vi "Drive Controller.vi"(8 "error in":errorcluster) -> ()   [LabVIEW 2020]
doc: "This VI executes continuously carrying out the current operation and responding to updates or new operation requests. It will often contain the timing or control code that is difficult to place directly in TeleOp. This VI generally opens all sensors and motors and isolates the rest of the robot code from knowing implementation details of how the operations are carried out."
uses:
  <vilib>/Rock Robotics/WPI/Framework/Completion Status.ctl
  Drive Setpoints.ctl
  Drive Operations.ctl
  <vilib>/Rock Robotics/WPI/SafetyOutput/WPI_SafetyOutputConfigMenu.ctl
  <vilib>/Rock Robotics/WPI/RobotDrive/WPI_RobotDriveOpen2MotorWithExistingMotors.vi
panel:
  in  "Interactive Values":T1
  in  "Buttons":cluster{"Execute Cmd":bool, "Abort Cmd":bool}
  out "Command Timing":cluster{"Start Time (ms)":u32, "Iterations":i32}
  out "Status":T3
  out "Setpoints":T4(graph)
  out "Current\nCmd":string
  # "Tip: The graph shows the motor setpoints. It may also be helpful to observe inputs and sensor values.\nYou may also want to display tuning or debugging controls."
  # "Interactive Command: You may fill in the settings for a command\nand schedule it with the Execute button. You can observe and abort\nany command while fine tuning the code for the controller."
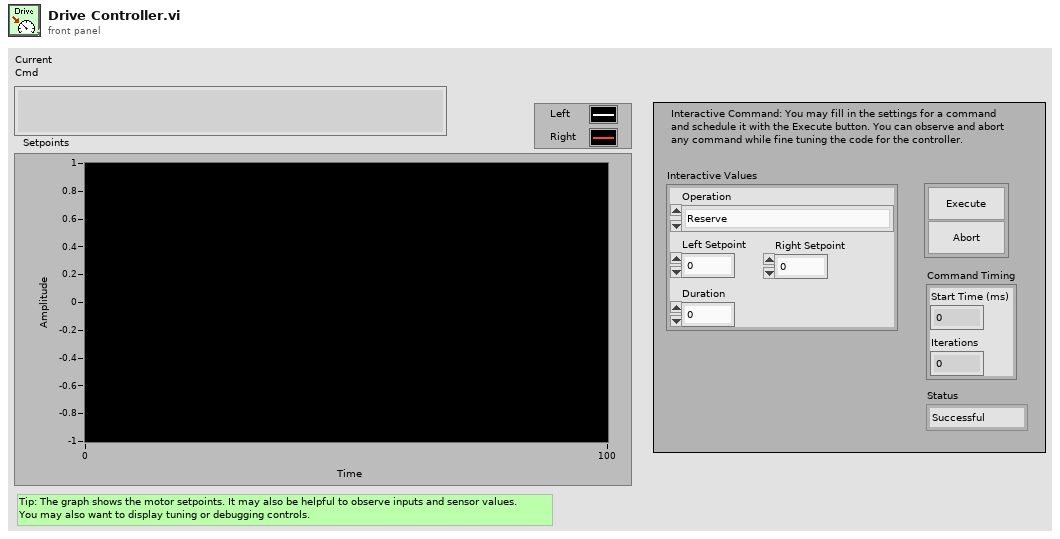
[diagram p1: front panel]
types:
  T1 = typedef "Drive Setpoints.ctl" = cluster{"Operation":T2, "Left Setpoint":dbl, "Right Setpoint":dbl, "Duration":dbl}
  T2 = typedef "Drive Operations.ctl" = enum16{"Reserve", "Read Current", "Immediate", "Drive for Time", "Drive for Distance"}
  T3 = typedef "Completion Status.ctl" = enum16{"Successful", "Aborted", "Incomplete"}
  T4 = cluster{"Left Setpoint":dbl, "Right Setpoint":dbl}
  T5 = typedef "WPI_SafetyOutputConfigMenu.ctl" = enum16{"Enable", "Disable"}
  T6 = typedef "WPI_MotorControlDeviceRef.ctl" = cluster{"DeviceStatus":errorcluster, "Type":T7, "PWM":cluster{"PWM Channel":T8, "DeadBand":T9}, "CAN":cluster{"Device Number":u8, "SetOutput VI Ref":variant, "GetOutput VI Ref":variant, "Enable VI Ref":variant, "Disable VI Ref":variant, "Data":variant}, "Invert":bool, "DIO PWM":cluster{"PWM \"Enable\" Channel":T8, "DIOChannel":T10, "PWM Rate":dbl}}
  T7 = typedef "WPI_MotorControlType.ctl" = enum16{"PWM", "CAN", "DIO PWM"}
  T8 = typedef "FPGA_DIOPWMChannel.ctl" = enum8{"PWM 0", "PWM 1", "PWM 2", "PWM 3", "PWM 4", "PWM 5", "PWM 6", "PWM 7", "PWM 8", "PWM 9", "PWM MXP 0", "PWM MXP 1", "PWM MXP 2", "PWM MXP 3", "PWM MXP 4", "PWM MXP 5", "PWM MXP 6", "PWM MXP 7", "PWM MXP 8", "PWM MXP 9", "Invalid"}
  T9 = typedef "WPI_PWMDeadband.ctl" = cluster{"Name":string, "maxPositivePwm":i32, "minPositivePwm":i32, "centerPwm":i32, "maxNegativePwm":i32, "minNegativePwm":i32, "angularRange":u16}
  T10 = typedef "FPGA_DIOChannel.ctl" = enum8{"DIO 0", "DIO 1", "DIO 2", "DIO 3", "DIO 4", "DIO 5", "DIO 6", "DIO 7", "DIO 8", "DIO 9", "DIO MXP 0", "DIO MXP 1", "DIO MXP 2", "DIO MXP 3", "DIO MXP 4", "DIO MXP 5", "DIO MXP 6", "DIO MXP 7", "DIO MXP 8", "DIO MXP 9", "DIO MXP 10", "DIO MXP 11", "DIO MXP 12", "DIO MXP 13", "DIO MXP 14", "DIO MXP 15", "SPI Port CS1", "SPI Port CS2", "SPI Port CS3", "SPI Port MISO", "SPI Port MOSI", "Invalid"}
  T11 = typedef "WPI_RobotDriveDevRef.ctl" = cluster{"DevStatus":errorcluster, "Motors[]":T6[], "Square Inputs":bool, "Max Output":dbl}
  T12 = typedef "Command Status Info.ctl" = cluster{"Name":string, "Status":T3, "notifier out":T13}
  T13 = typedef "Completion Notifier.ctl" = refnum<notifier>
  T14 = cluster{"SubSystem Data":T1, cluster{"Start Time (ms)":u32, "Iterations":i32}, cluster{"Command Info":T12, "Description":string, "Default Command":T1, "queue out":refnum<queue>, "Subsystem Name":string}}
  T15 = cluster{"SubSystem Data":T1, cluster{"Start Time (ms)":u32, "Iterations":i32}, "Default Command Arguments":cluster{"Command Info":T12, "Description":string, "Default Command":T1, "queue out":refnum<queue>, "Subsystem Name":string}}
  T16 = cluster{"Don't move motors while reserved":dbl, "Don't move motors while reserved":dbl}
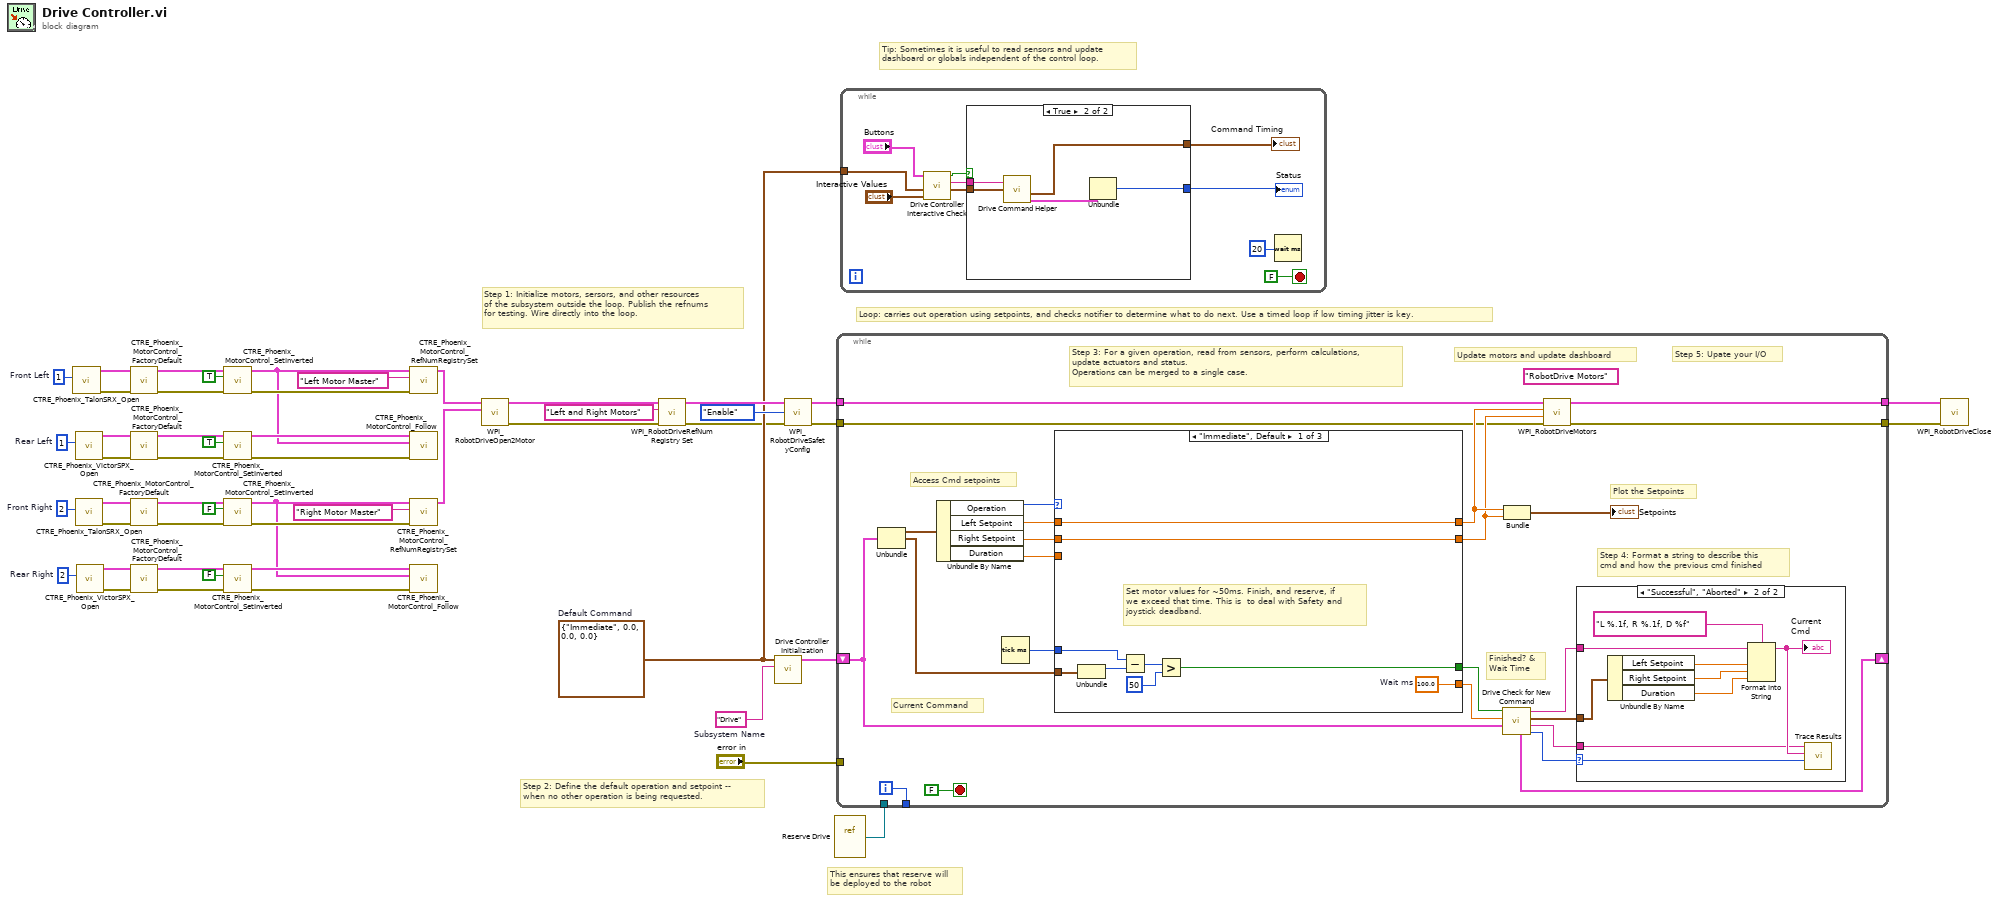
[diagram p0: block diagram]
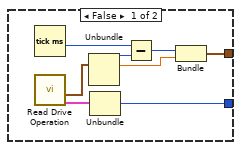
[diagram p2: hidden frame]
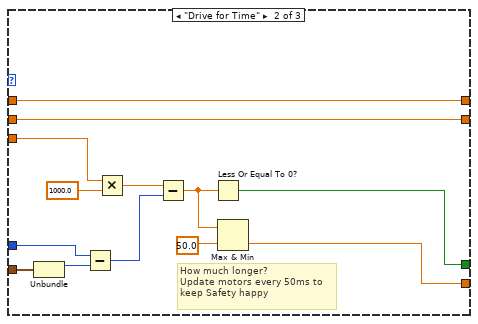
[diagram p4: hidden frame]
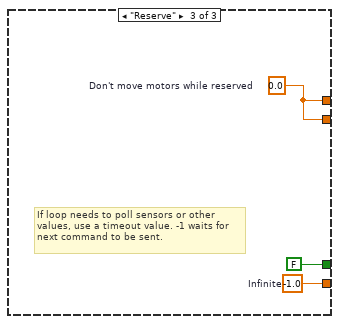
[diagram p5: hidden frame]
diagram:
  w18 = u8 2  # Rear Right
  w19 = u8 2  # Front Right
  w20 = u8 1  # Rear Left
  w21 = u8 1  # Front Left
  w43 = T1 {"Operation"=enum."Immediate", "Left Setpoint"=0.0, "Right Setpoint"=0.0, "Duration"=0.0}  # Default Command
  w51 = "Drive"  # Subsystem Name
  # "This ensures that reserve will\nbe deployed to the robot"
  # "Tip: Sometimes it is useful to read sensors and update\ndashboard or globals independent of the control loop."
  # "Step 2: Define the default operation and setpoint --\nwhen no other operation is being requested."
  # "Step 1: Initialize motors, sersors, and other resources\nof the subsystem outside the loop. Publish the refnums\nfor testing. Wire directly into the loop."
  # "Loop: carries out operation using setpoints, and checks notifier to determine what to do next. Use a timed loop if low timing jitter is key."
  n1 = call <vilib>:"CTRE_Phoenix_TalonSRX_Open.vi"("Device Number"=w21) -> ("error out"=w38:errorcluster, "PhoenixMotorControlDevRef"=w42:T6)  [unwired: 9 in]
  n2 = call <vilib>:"CTRE_Phoenix_VictorSPX_Open.vi"("Device Number"=w20) -> ("error out"=w35:errorcluster, "PhoenixMotorControlDevRef"=w40:T6)  [unwired: 9 in]
  n3 = call <vilib>:"CTRE_Phoenix_TalonSRX_Open.vi"("Device Number"=w19) -> ("error out"=w27:errorcluster, "PhoenixMotorControlDevRef"=w32:T6)  [unwired: 9 in]
  n4 = call <vilib>:"CTRE_Phoenix_VictorSPX_Open.vi"("Device Number"=w18) -> ("error out"=w24:errorcluster, "PhoenixMotorControlDevRef"=w30:T6)  [unwired: 9 in]
  n5 = call <vilib>:"CTRE_Phoenix_MotorControl_FactoryDefault.vi"("error in"=w38, "PhoenixMotorControlDevRef"=w42) -> ("error out"=w37:errorcluster, "PhoenixMotorControlDevRef"=w41:T6)  [unwired: 8 in]
  n6 = call <vilib>:"CTRE_Phoenix_MotorControl_FactoryDefault.vi"("error in"=w35, "PhoenixMotorControlDevRef"=w40) -> ("error out"=w34:errorcluster, "PhoenixMotorControlDevRef"=w39:T6)  [unwired: 8 in]
  n7 = call <vilib>:"CTRE_Phoenix_MotorControl_FactoryDefault.vi"("error in"=w27, "PhoenixMotorControlDevRef"=w32) -> ("error out"=w26:errorcluster, "PhoenixMotorControlDevRef"=w31:T6)  [unwired: 8 in]
  n8 = call <vilib>:"CTRE_Phoenix_MotorControl_FactoryDefault.vi"("error in"=w24, "PhoenixMotorControlDevRef"=w30) -> ("error out"=w23:errorcluster, "PhoenixMotorControlDevRef"=w29:T6)  [unwired: 8 in]
  n9 = call <vilib>:"CTRE_Phoenix_MotorControl_SetInverted.vi"("error in (no error)"=w37, "Invert?"=TRUE, "PhoenixMotorControlDevRef"=w41) -> ("error out"=w36:errorcluster, "PhoenixMotorControlDevRef"=w12:T6)  [unwired: 7 in]
  n10 = call <vilib>:"CTRE_Phoenix_MotorControl_SetInverted.vi"("error in (no error)"=w34, "Invert?"=TRUE, "PhoenixMotorControlDevRef"=w39) -> ("error out"=w33:errorcluster, "PhoenixMotorControlDevRef"=w17:T6)  [unwired: 7 in]
  n11 = call <vilib>:"CTRE_Phoenix_MotorControl_SetInverted.vi"("error in (no error)"=w26, "Invert?"=FALSE, "PhoenixMotorControlDevRef"=w31) -> ("error out"=w25:errorcluster, "PhoenixMotorControlDevRef"=w11:T6)  [unwired: 7 in]
  n12 = call <vilib>:"CTRE_Phoenix_MotorControl_SetInverted.vi"("error in (no error)"=w23, "Invert?"=FALSE, "PhoenixMotorControlDevRef"=w29) -> ("error out"=w22:errorcluster, "PhoenixMotorControlDevRef"=w28:T6)  [unwired: 7 in]
  n13 = call <vilib>:"CTRE_Phoenix_MotorControl_RefNumRegistrySet.vi"("error in (no error)"=w36, "refnum name"="Left Motor Master", "PhoenixMotorControlDevRef"=w12) -> ("PhoenixMotorControlDevRef"=w9:T6)  [unwired: 7 in, 1 out]
  n14 = call <vilib>:"CTRE_Phoenix_MotorControl_Follow.vi"("error in (no error)"=w33, "Master Controller to Follow"=w12, "PhoenixMotorControlDevRef"=w17) -> ()  [unwired: 7 in, 2 out]
  n15 = call <vilib>:"CTRE_Phoenix_MotorControl_RefNumRegistrySet.vi"("error in (no error)"=w25, "refnum name"="Right Motor Master", "PhoenixMotorControlDevRef"=w11) -> ("PhoenixMotorControlDevRef"=w8:T6)  [unwired: 7 in, 1 out]
  n16 = call <vilib>:"CTRE_Phoenix_MotorControl_Follow.vi"("error in (no error)"=w22, "Master Controller to Follow"=w11, "PhoenixMotorControlDevRef"=w28) -> ()  [unwired: 7 in, 2 out]
  n17 = call-poly <vilib>:"WPI_RobotDriveOpen2Motor.vi"("Right Motor Dev Ref"=w8, "Left Motor Dev Ref"=w9) -> ("error out"=w5:errorcluster, "RobotDriveDevRef"=w10:T11)  [unwired: 3 in, 5 out]
  n18 = call <vilib>:"WPI_RobotDriveRefNum Registry Set.vi"("error in (no error)"=w5, "refnum name"="Left and Right Motors", "RobotDriveDevRef"=w10) -> ("error out"=w4:errorcluster, "RobotDriveDevRef"=w49:T11)  [unwired: 1 in, 6 out]
  n19 = call "Drive Controller Initialization.vi"("Subsystem Name"=w51, "Default Command"=w43) -> ("Current Command"=w45:T14)  [unwired: 9 in]
  n20 = call <vilib>:"WPI_RobotDriveSafetyConfig.vi"("error in (no error)"=w4, "mode"=WPI_SafetyOutputConfigMenu."Enable", "RobotDriveDevRef"=w49) -> ("error out"=w3:errorcluster, "RobotDriveDevRef"=w47:T11)  [unwired: 7 in]
  n21 = vi-ref "Reserve Drive.vi"() -> (w44:refnum<vi>)
  n22 = while {
    shift-right: [w62] -> _
    shift-left: w45 -> [w55]
    tunnel: [w74] -> _
    tunnel: w47 -> [w70]
    tunnel: "error in" -> [_]
    tunnel: w44 -> [_]
    tunnel: w3 -> [w54]
    tunnel: [w53] -> w2
    tunnel: [w52] -> w1
    i -> [w74]
    stop <- FALSE stop-if-true
    (unwired) "RobotDrive Motors" ("Name")
    # "Step 5: Upate your I/O"
    # "Step 4: Format a string to describe this\ncmd and how the previous cmd finished"
    # "Current Command"
    # "Update motors and update dashboard"
    # "Plot the Setpoints"
    # "Access Cmd setpoints"
    # "Finished? &\nWait Time"
    # "Step 3: For a given operation, read from sensors, perform calculations,\nupdate actuators and status.\nOperations can be merged to a single case."
    n23 = Unbundle(w55) -> ("SubSystem Data"=w69:T1, w56:cluster{"Start Time (ms)":u32, "Iterations":i32})  [unwired: 1 out]
    n24 = Unbundle By Name(w69) -> ("Operation"=w68:T2, "Left Setpoint"=w67:dbl, "Right Setpoint"=w66:dbl, "Duration"=w65:dbl)
    n25 = Tick Count (ms)() -> (millisecond timer value=w64:u32)
    n26 = case shown="\"Immediate\", Default" w68 {
      tunnel: [w93 w94 w109] -> w61
      tunnel: [w86 w101 FALSE ("ignore previous (F)")] -> w60
      tunnel: w56 -> [w85 w103 _]
      tunnel: [w92 w100 w107] -> w72
      tunnel: [w91 w99 w107] -> w71
      tunnel: w67 -> [w92 w100 _]
      tunnel: w66 -> [w91 w99 _]
      tunnel: w65 -> [_ w98 _]
      tunnel: w64 -> [w87 w97 _]
      frame "Immediate", Default {
        w93 = 100.0  # Wait ms
        # "Set motor values for ~50ms. Finish, and reserve, if\nwe exceed that time. This is  to deal with Safety and\njoystick deadband."
        n27 = Unbundle(w85) -> ("Start Time (ms)"=w88:u32)  [unwired: 1 out]
        n28 = Subtract(x=w87, y=w88) -> (x-y=w89:u32)
        n29 = Greater?(x=w89, y=u8 50 ("Left Motor")) -> (0:w86:bool)
      }
      frame "Drive for Time" {
        # "How much longer?\nUpdate motors every 50ms to\nkeep Safety happy"
        n30 = Unbundle(w103) -> ("Start Time (ms)"=w102:u32)  [unwired: 1 out]
        n31 = Subtract(x=w97, y=w102) -> (x-y=w106:u32)
        n32 = Multiply(x=w98, y=1000.0) -> (x*y=w105:dbl)
        n33 = Subtract(x=w105, y=w106) -> (x-y=w96:dbl)
        n34 = Less Or Equal To 0?(x=w96) -> (x <= 0?=w101:bool)
        n35 = Max & Min(x=w96, y=50.0) -> (min(x,y)=w94:dbl)  [unwired: 1 out]
      }
      frame "Reserve" {
        w107 = 0.0  # Don't move motors while reserved
        w109 = -1.0  # Infinite
        # "If loop needs to poll sensors or other\nvalues, use a timeout value. -1 waits for\nnext command to be sent."
      }
    }
    n36 = call "Drive Check for New Command.vi"("input cluster"=w55, "Wait time (ms)"=w61, "Finished?"=w60) -> ("Completion"=w63:T3, "Subsystem Name"=w57:string, "Current Command"=w58:T1, "Initial Trace String"=w59:string, "Next Command"=w62:T15)  [unwired: 4 in]
    n37 = Bundle("Don't move motors while reserved"=w72, "Don't move motors while reserved"=w71) -> (→"Setpoints":T16)  [unwired: 1 in]
    n38 = call <vilib>:"WPI_RobotDriveMotors.vi"("error in (no error)"=w54, "RightSpeed"=w71, "LeftSpeed"=w72, "RobotDriveDevRef"=w70) -> ("error out"=w52:errorcluster, "RobotDriveDevRef"=w53:T11)  [unwired: 6 out]
    n39 = case shown="\"Successful\", \"Aborted\"" w63 {
      selector: w63 -> [_ w84]
      tunnel: w59 -> [_ w79]
      tunnel: w58 -> [_ w80]
      tunnel: w57 -> [_ w76]
      frame "Incomplete", Default {
        # "Continuing current command"
      }
      frame "Successful", "Aborted" {
        # "Report and setup for next command"
        n40 = Unbundle By Name(w80) -> ("Left Setpoint"=w82:dbl, "Right Setpoint"=w83:dbl, "Duration"=w77:dbl)
        n41 = Format Into String(format string="L %.1f, R %.1f, D %f", initial string=w79, w82, w83, w77) -> (resulting string=w78:string)  [unwired: 1 in, 1 out]
        "Current\nCmd" <- w78
        n42 = call <vilib>:"Trace Results.vi"("Status of previous command"=w84, "Description"=w78, "Subsystem"=w76) -> ()  [unwired: 9 in]
      }
    }
  }
  n43 = while {
    tunnel: w43 -> [w111]
    stop <- FALSE stop-if-true
    n44 = call "Drive Controller Interactive Check.vi"("Interactive Command In"="Interactive Values", "Default Command"=w111, "Buttons"="Buttons") -> ("Interactive Command Out"=w113:T1, "Trace String"=w114:string, "Schedule"=w115:bool)  [unwired: 6 in]
    n45 = case shown="True" w115 {
      tunnel: [w124 w132] -> w116
      tunnel: [w123 w128] -> w117
      tunnel: w114 -> [_ w130]
      tunnel: w113 -> [_ w129]
      frame False {
        n46 = Tick Count (ms)() -> (millisecond timer value=w127:u32)
        n47 = call "Read Drive Operation.vi"() -> ("Command Info"=w121:T12, "SubSystem Data"=w120:T1)  [unwired: 9 in, 1 out]
        n48 = Unbundle(w120) -> ("Operation"=w125:T2, "Left Setpoint"=w122:dbl)  [unwired: 2 out]
        n49 = Unbundle(w121) -> ("Status"=w124:T3)  [unwired: 2 out]
        n50 = Subtract(x=w127, y=w125) -> (x-y=w126:u32)
        n51 = Bundle(w126, "Left Setpoint"=w122) -> (w123:cluster{u32, "Left Setpoint":dbl})  [unwired: 1 in]
      }
      frame True {
        n52 = call "Drive Command Helper.vi"("Description"=w130, "SubSystem Data"=w129) -> ("Command Info Out"=w131:T12, "Command Timing"=w128:cluster{"Start Time (ms)":u32, "Iterations":i32})  [unwired: 7 in, 1 out]
        n53 = Unbundle(w131) -> ("Status"=w132:T3)  [unwired: 2 out]
      }
    }
    "Status" <- w116
    "Command Timing" <- w117
    n54 = Wait (ms)(milliseconds to wait=u32 20) -> ()  [unwired: 1 out]
  }
  n55 = call <vilib>:"WPI_RobotDriveClose.vi"("error in (no error)"=w1, "RobotDriveDevRef"=w2) -> ()  [unwired: 9 in, 1 out]
